vi "SendSoftwareTrigger.vi"(8 "error in (no error)":errorcluster, 11 "ScopeBase In":refnum<class "ScopeBase.lvclass">) -> (0 "error out":errorcluster, 3 "ScopeBase Out":refnum<class "ScopeBase.lvclass">)   [LabVIEW 2018, in "ScopeBase.lvclass"]
uses:
  ScopeBase.lvclass
  ScopeBase.lvclass/ScopeBase.ctl
  <vilib>/Utility/error.llb/Error Cluster From Error Code.vi
  <vilib>/rvi/errors/niLvFpgaAdjustHostInterfaceError.vi
  <vilib>/rvi/interface/nirviReadWriteControl/nirviReadWriteControl.xnode
  FpgaRef/FpgaRefBase/Common FPGA ref.ctl
  FpgaRef/FpgaRefBase/FpgaRefBase.lvclass
  NiFpgaLv.dll
  <vilib>/rvi/interface/Simulation/niFpgaSimulationCallBeginRW.vi
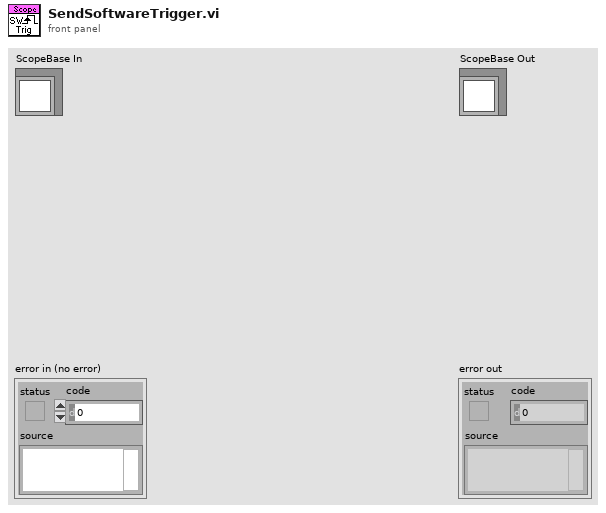
[diagram p1: front panel]
types:
  T1 = typedef "5782_trigger_type.ctl" = enum16{"Software", "Trigger input"}
  T2 = typedef "Common FPGA ref.ctl" = refnum<k20>
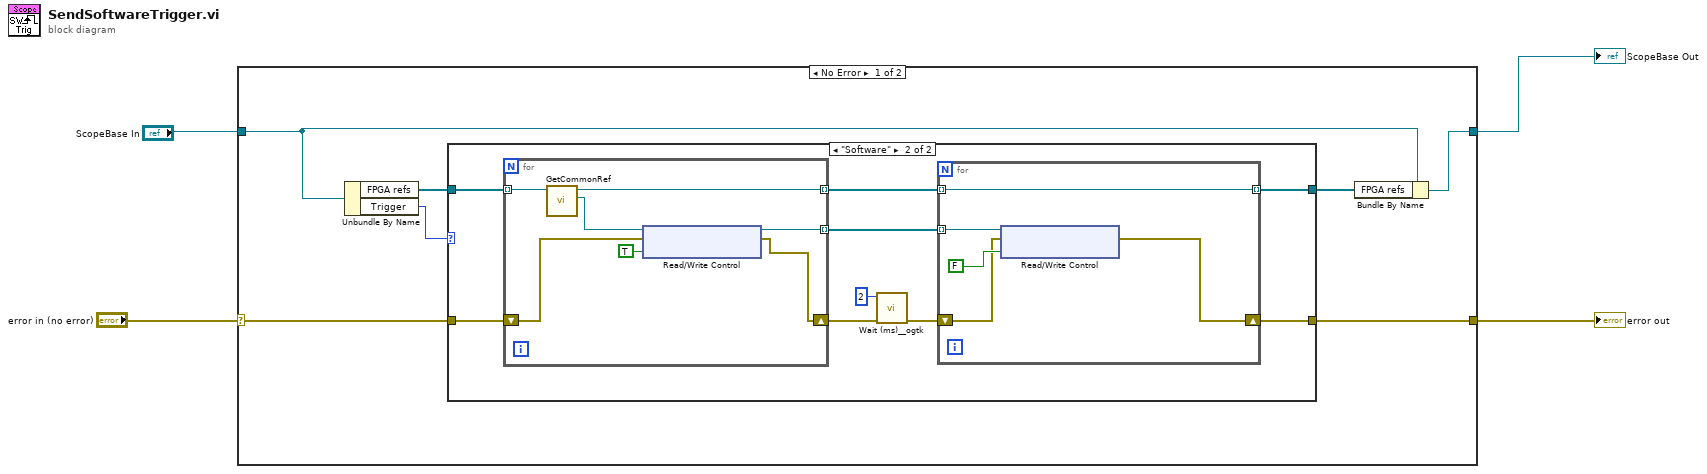
[diagram p0: block diagram]
diagram:
  n1 = case shown="No Error" "error in (no error)" {
    selector: "error in (no error)" -> [w6 w35]
    tunnel: [w9 w36] -> w2
    tunnel: "ScopeBase In" -> [w8 w36]
    tunnel: [w5 w35] -> w1
    frame No Error {
      n2 = Unbundle By Name(w8) -> ("FPGA refs"=w11:refnum<class "FpgaRefBase.lvclass">[], "Trigger"=w7:T1)
      n3 = case shown="\"Software\"" w7 {
        tunnel: w11 -> [w13 w22]
        tunnel: [w13 w15] -> w10
        tunnel: w6 -> [w12 w21]
        tunnel: [w12 w14] -> w5
        frame Default {
        }
        frame "Software" {
          n4 = for {
            tunnel: w22 -> [w33] mode=indexing
            tunnel: [w34] -> w20 mode=indexing
            shift-right: [w29] -> w18
            shift-left: w21 -> [w30]
            tunnel: [w28] -> w17 mode=indexing
            n5 = call-dynamic "GetCommonRef.vi"("FpgaRefBase in"=w33) -> ("Common ref"=w31:T2, "FpgaRefBase out"=w34:refnum<class "FpgaRefBase.lvclass">)  [unwired: 8 in, 1 out]
            n6 = xnode "Read/Write Control"("FPGA VI Reference In"=w31, "error in"=w30, "Trigger Acquisition"=TRUE) -> ("FPGA VI Reference Out"=w28:T2, "error out"=w29:errorcluster)
          }
          n7 = call <userlib>:"Wait (ms)__ogtk.vi"("error in (no error)"=w18, "milliseconds to wait"=u32 2) -> ("error out"=w16:errorcluster)  [unwired: 8 in, 1 out]
          n8 = for {
            tunnel: w20 -> [w24] mode=indexing
            tunnel: w17 -> [w26] mode=indexing
            tunnel: [w24] -> w15 mode=indexing
            shift-right: [w23] -> w14
            shift-left: w16 -> [w25]
            n9 = xnode "Read/Write Control"("FPGA VI Reference In"=w26, "error in"=w25, "Trigger Acquisition"=FALSE) -> ("error out"=w23:errorcluster)  [unwired: 1 out]
          }
        }
      }
      n10 = Bundle By Name(cluster=w8, "FPGA refs"=w10) -> (w9:refnum<class "ScopeBase.lvclass">)
    }
    frame Error {
    }
  }
  "error out" <- w1
  "ScopeBase Out" <- w2
